vi "sync.vi"(8 "error in (no error)":errorcluster, 11 "5785_2_x_1600MHz in":refnum<class "5785_2_x_1600MHz.lvclass">) -> (0 "error out":errorcluster, 3 "5785_2_x_1600MHz out":refnum<class "5785_2_x_1600MHz.lvclass">)   [LabVIEW 2021, in "5785_2_x_1600MHz.lvclass"]
uses:
  5785_2_x_1600MHz.lvclass
  5785_2_x_1600MHz.lvclass/5785_2_x_1600MHz.ctl
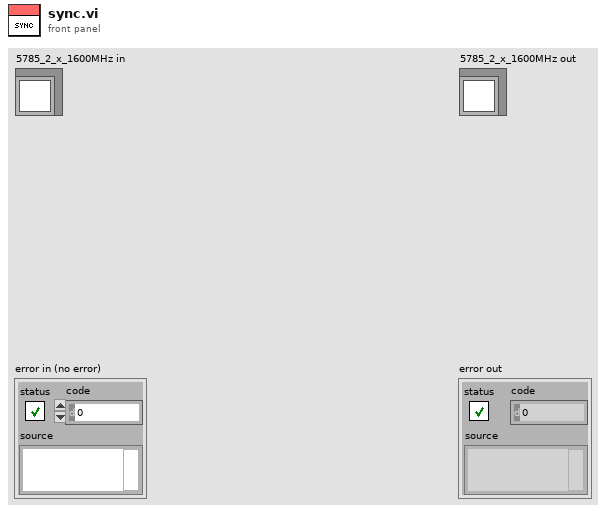
[diagram p1: front panel]
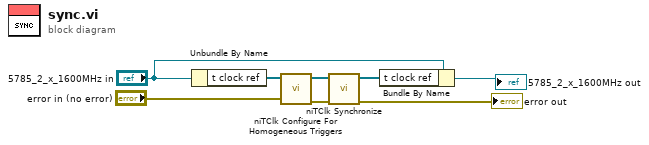
[diagram p0: block diagram]
diagram:
  n1 = Unbundle By Name("5785_2_x_1600MHz in") -> ("t clock ref"=w4:refnum<k20>[])
  n2 = call <instrlib>:"niTClk Configure For Homogeneous Triggers.vi"("error in (no error)"="error in (no error)", "sessions"=w4) -> ("error out"=w5:errorcluster, "sessions out"=w6:refnum<k20>[])  [unwired: 8 in]
  n3 = call <instrlib>:"niTClk Synchronize.vi"("error in (no error)"=w5, "sessions"=w6) -> ("error out"=→"error out":errorcluster, "sessions out"=w3:refnum<k20>[])  [unwired: 8 in]
  n4 = Bundle By Name(cluster="5785_2_x_1600MHz in", "t clock ref"=w3) -> (→"5785_2_x_1600MHz out":refnum<class "5785_2_x_1600MHz.lvclass">)
